vi "Search Virtual Folders (DFS Main).vi"(8 "Error In":errorcluster, 10 "Filename (including file extension)":string, 11 "Library Ref":refnum<vi>) -> (0 "Error Out":errorcluster)   [LabVIEW 2022 SP3]
doc: "<add documentation here>"
uses:
  DFS States (enum).ctl
panel:
  out "Virtual Folder Path (index 0 is top-level folder)":string[](array[string])
  out "File found inside a virtual folder?":bool
  # "Development\nControls or indicators that are useful for development or testing, but which are not outputs of the VI."
  # "Input\nInputs to the VI"
  # "Output\nOutputs of the VI"
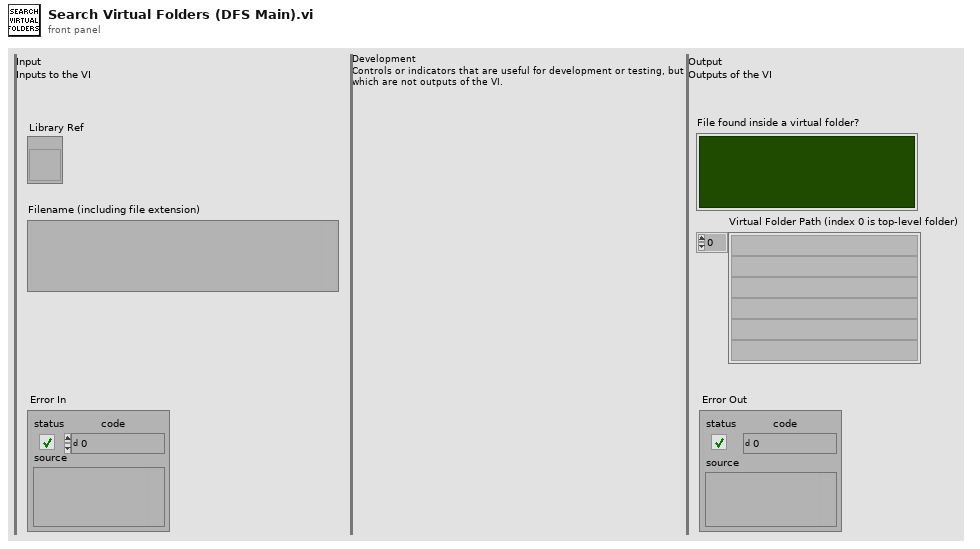
[diagram p1: front panel]
types:
  T1 = typedef "DFS States (enum).ctl" = enum16{"Init", "Exit"}
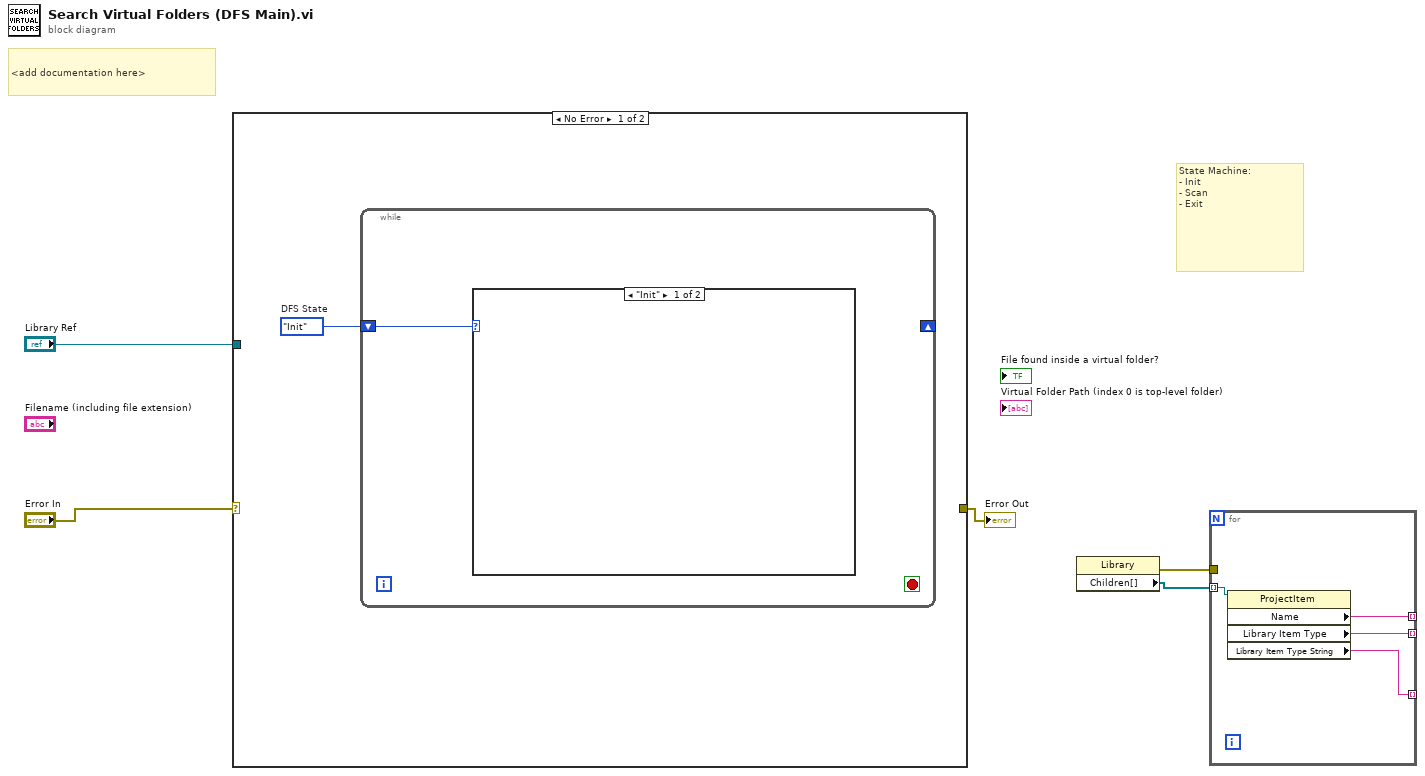
[diagram p0: block diagram]
diagram:
  # "State Machine:\n- Init\n- Scan\n- Exit"
  # "<add documentation here>"
  n1 = case shown="No Error" "Error In" {
    selector: "Error In" -> [_ w8]
    tunnel: [_ w8] -> w4
    tunnel: "Library Ref" -> [_ _]
    frame No Error {
      w6 = DFS_States_(enum)."Init"  # DFS State
      n2 = while {
        shift-right: _ -> [_]
        shift-left: w6 -> [w7]
        stop <- _ stop-if-true
        n3 = case shown="\"Init\"" w7 {
          frame "Init" {
          }
          frame "Exit" {
          }
        }
      }
    }
    frame Error {
    }
  }
  "Error Out" <- w4
  n4 = property class="Library"() -> (error out=w2:errorcluster, "Children[]"=w1:refnum<vi>[])  [unwired: 2 in, 1 out]
  n5 = for {
    tunnel: w1 -> [w12] mode=indexing
    tunnel: [w11] -> _ mode=indexing
    tunnel: [w10] -> _ mode=indexing
    tunnel: [w9] -> _ mode=indexing
    tunnel: w2 -> [_]
    n6 = property class="ProjectItem"(reference=w12) -> ("Name"=w11:string, "Library Item Type"=w10:string, "Library Item Type String"=w9:string)  [unwired: 1 in, 2 out]
  }
